vi "Dashboard Main.vi"() -> ()   [LabVIEW 2012]
uses:
  <vilib>/Utility/config.llb/Read Key (String).vi
  <vilib>/Utility/config.llb/Read Key (I32).vi
  <vilib>/Utility/config.llb/Write Key (String).vi
  <vilib>/Utility/config.llb/Write Key (I32).vi
  <vilib>/Utility/config.llb/NI_LVConfig.lvlib
panel:
  in  "?":bool
  out "Camera Image 2":T1(plugin-control)
  out "Mbps":dbl format="%#.1g"
  in  "Enable":bool
  in  "DB Camera Config":bool
  out "Mbps 2":bool
  out "fps":dbl format="%#.1g"
  out "Camera Image":T1(plugin-control)
  out "Battery Value":dbl(slide) scale=0.0..14.0 scale format="%#_2e"
  out "Battery":sgl(graph)
  in  "Camera Settings":T2={"Frate Rate"=30, "Compression"=30, "Size"=1} {"Frate Rate" scale=1.0..30.0; "Size" items=["640x480", "320x240", "160x120"]}
  out "Mode":T3(ring)=enum."Auto Disabled"
  out "Robot IP":string
  # "Robot IP:"
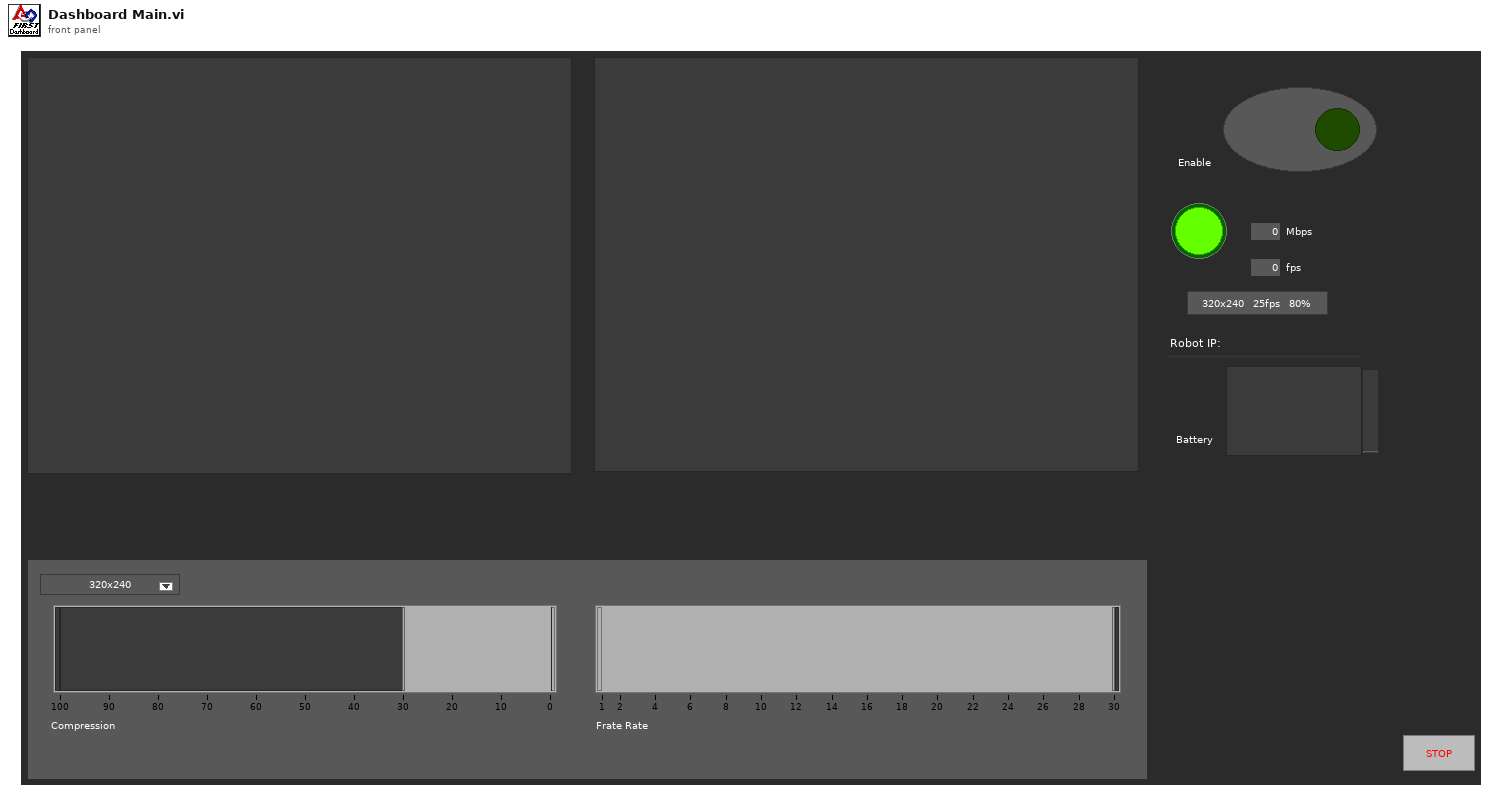
[diagram p1: front panel]
types:
  T1 = typedef "IMAQ Image.ctl" = refnum<image>
  T2 = cluster{"Frate Rate":i32, "Compression":i32, "Size":u16}
  T3 = enum8{"Tele-Op Disabled", "Tele-Op Enabled", "Auto Disabled", "Auto Enabled", "Test Disabled", "Test Enabled", ""}
  T4 = typedef "Image Type" = u32
  T5 = typedef "LVRectTypeDef.ctl" = cluster{"Left":i16, "Top":i16, "Right":i16, "Bottom":i16}
  T6 = cluster{"Competition mode":bool, "Robot Link":bool, "Autonomous":bool, "Enabled":bool, "E-Stop":bool, "Simulated":bool, "TestMode":bool, "Docked Window":bool}
  T7 = typedef "NI_LVConfig.lvlib/Config Data RefNum.ctl" = refnum<k1>
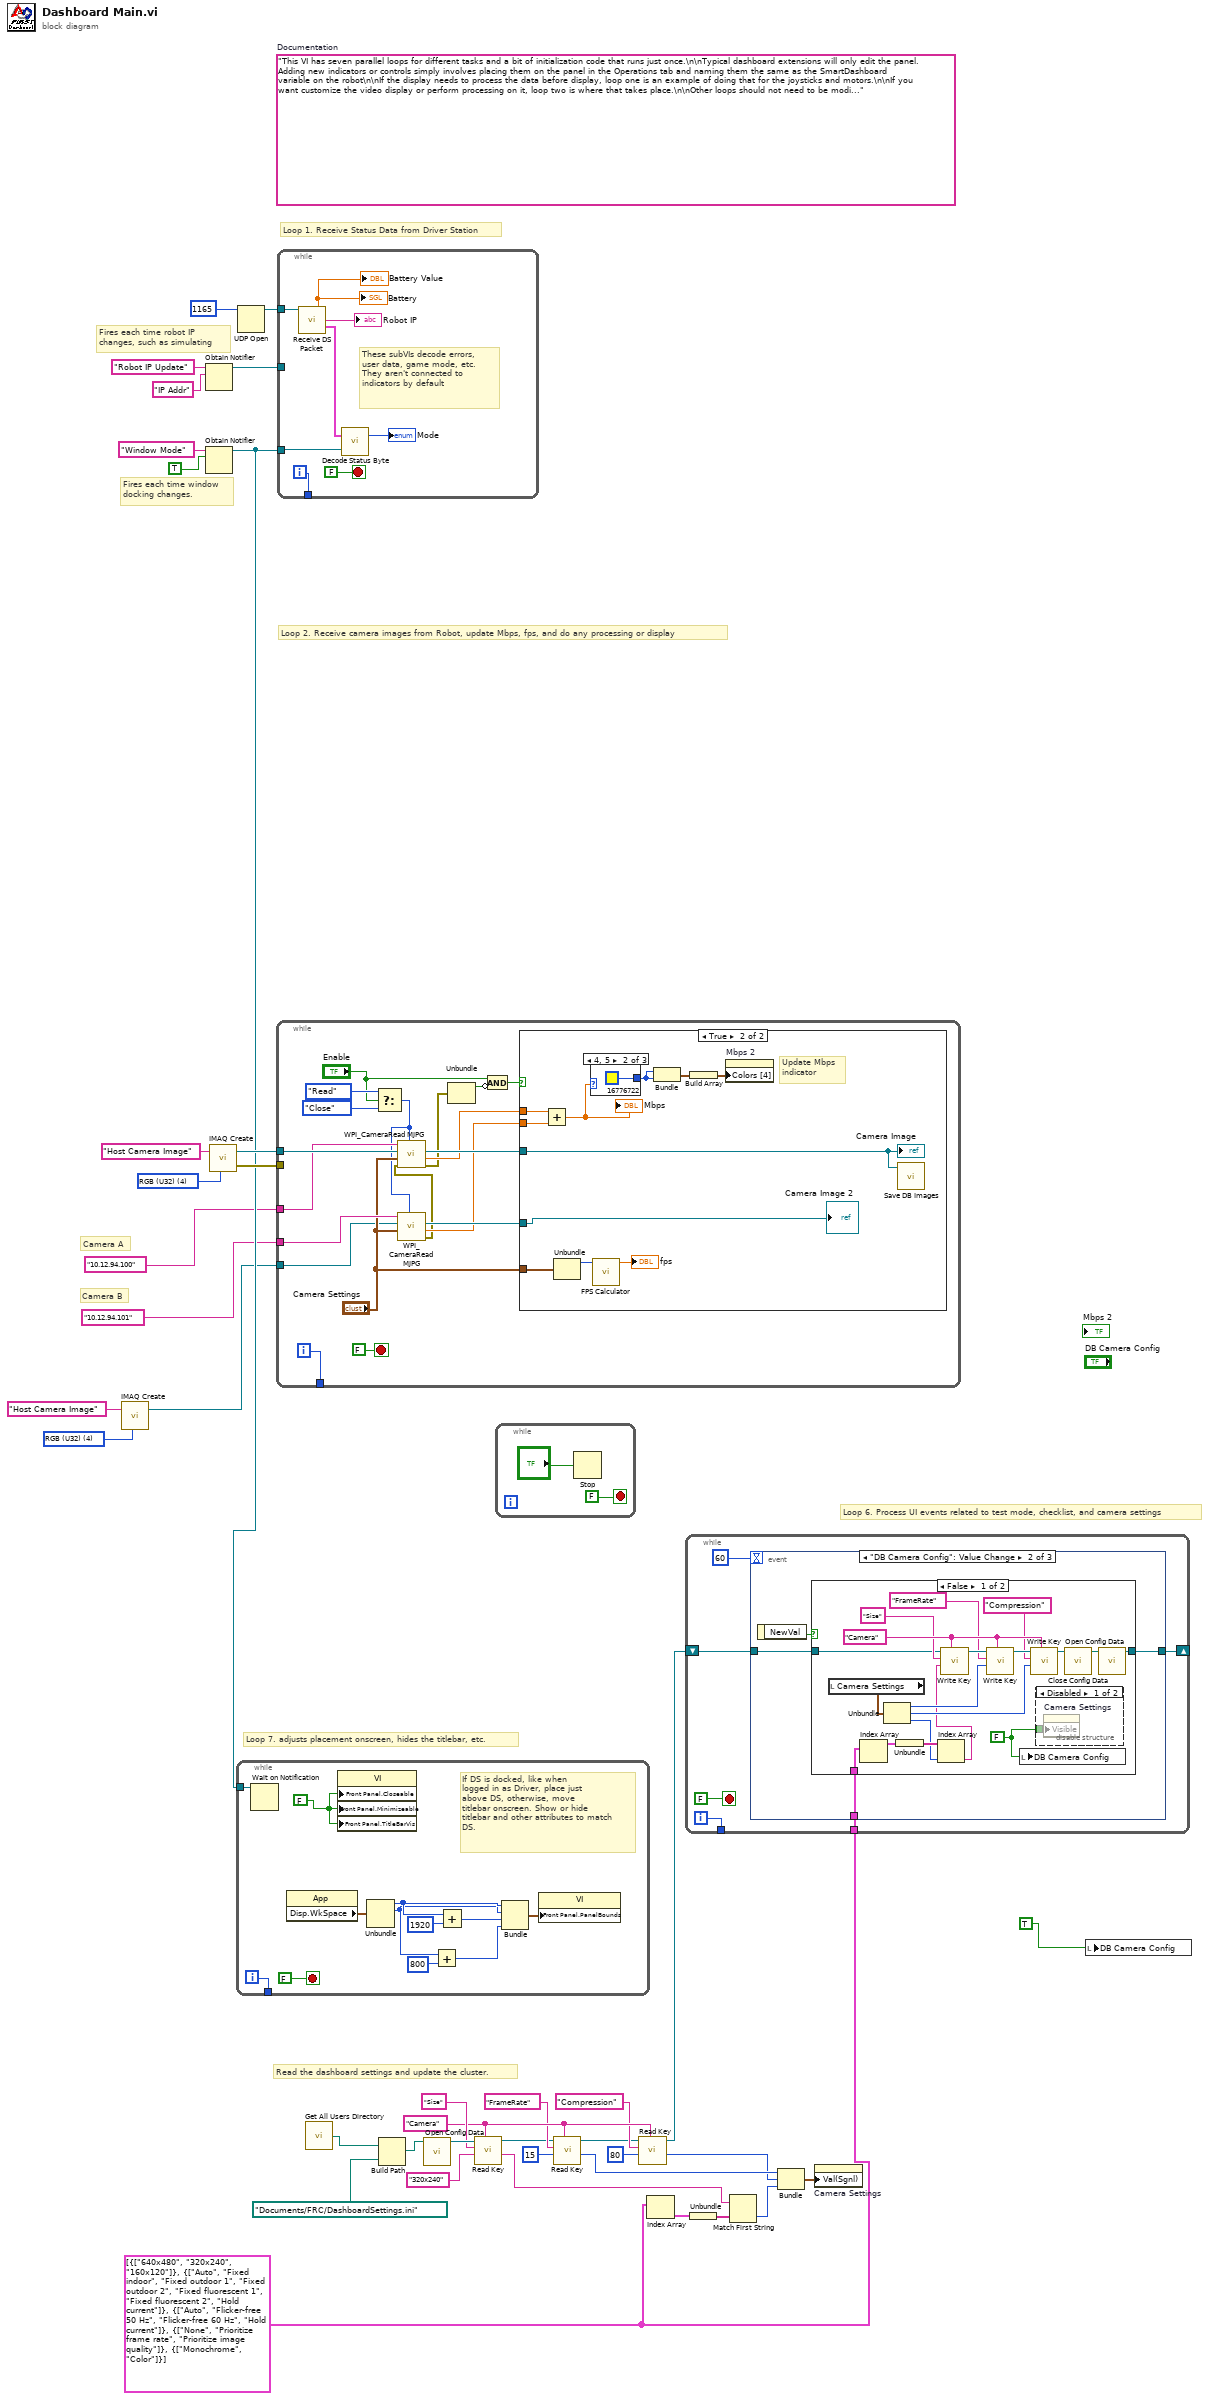
[diagram p0: block diagram]
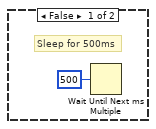
[diagram p2: hidden frame]
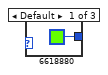
[diagram p3: hidden frame]
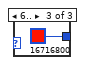
[diagram p4: hidden frame]
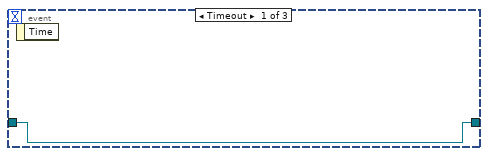
[diagram p5: hidden frame]
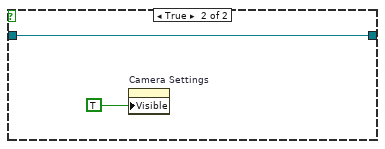
[diagram p7: hidden frame]
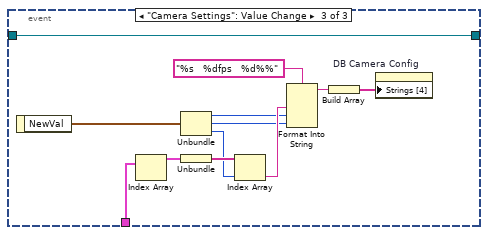
[diagram p8: hidden frame]
diagram:
  w3 = T4 4 items=["Grayscale (U8)", "Grayscale (I16)", "Grayscale (SGL)", "Complex (CSG)", "RGB (U32)", "HSL (U32)", "RGB (U64)"] ("Image Type")
  w22 = "Camera"
  w14 = cluster{string[]}[] [{["640x480", "320x240", "160x120"]}, {["Auto", "Fixed indoor", "Fixed outdoor 1", "Fixed outdoor 2", "Fixed fluorescent 1", "Fixed fluorescent 2", "Hold current"]}, {["Auto", "Flicker-free 50 Hz", "Flicker-free 60 Hz", "Hold current"]}, {["None", "Prioritize frame rate", "Prioritize image quality"]}, {["Monochrome", "Color"]}]
  (unwired) "This VI has seven parallel loops for different tasks and a bit of initialization code that runs just once.\n\nTypical dashboard extensions will only edit the panel. Adding new indicators or controls simply involves placing them on the panel in the Operations tab and naming them the same as the SmartDashboard variable on the robot\n\nIf the display needs to process the data before display, loop one is an example of doing that for the joysticks and motors.\n\nIf you want customize the video display or perform processing on it, loop two is where that takes place.\n\nOther loops should not need to be modified. They are pretty standard, and document the task they perform."  # Documentation
  w38 = T4 4 items=["Grayscale (U8)", "Grayscale (I16)", "Grayscale (SGL)", "Complex (CSG)", "RGB (U32)", "HSL (U32)", "RGB (U64)"] ("Image Type")
  # "Camera B"
  # "Camera A"
  # "Fires each time robot IP\nchanges, such as simulating"
  # "Fires each time window\ndocking changes."
  # "Loop 6. Process UI events related to test mode, checklist, and camera settings"
  # "Read the dashboard settings and update the cluster."
  # "Loop 7. adjusts placement onscreen, hides the titlebar, etc."
  # "Loop 1. Receive Status Data from Driver Station"
  # "Loop 2. Receive camera images from Robot, update Mbps, fps, and do any processing or display"
  n1 = call "IMAQ Create"("Image Name"="Host Camera Image", "Image Type"=w3) -> ("New Image"=w1:T1)  [unwired: 2 in, 2 out]
  n2 = Obtain Notifier(name (unnamed)="Robot IP Update", notification data type="IP Addr" ("name (unnamed)")) -> (notifier out=w32:refnum<notifier>)  [unwired: 2 in, 2 out]
  n3 = Obtain Notifier(name (unnamed)="Window Mode", notification data type=TRUE) -> (notifier out=w29:refnum<notifier>)  [unwired: 2 in, 2 out]
  n4 = call "IMAQ Create"("Image Name"="Host Camera Image", "Image Type"=w38) -> ("New Image"=w36:T1, "error out"=w35:errorcluster)  [unwired: 2 in, 1 out]
  n5 = while {
    tunnel: w29 -> [w51]
    tunnel: [w50] -> _
    i -> [w50]
    stop <- FALSE stop-if-true
    w41 = FALSE ("Front Panel Window:Closeable")
    # "If DS is docked, like when\nlogged in as Driver, place just\nabove DS, otherwise, move\ntitlebar onscreen. Show or hide\ntitlebar and other attributes to match\nDS."
    n6 = Wait on Notification(notifier=w51) -> ()  [unwired: 3 in, 4 out]
    n7 = property class="App"() -> ("Disp.WkSpace"=w43:T5)  [unwired: 2 in, 2 out]
    n8 = property class="VI"("Front Panel.Closeable"=w41, "Front Panel.Minimizeable"=w41, "Front Panel.TitleBarVis"=w41) -> ()  [unwired: 2 in, 2 out]
    n9 = Unbundle(w43) -> ("Left"=w49:i16, "Top"=w48:i16)  [unwired: 2 out]
    n10 = Add(x=w48, y=i16 800) -> (x+y=w45:i16)
    n11 = Add(x=w49, y=i16 1920) -> (x+y=w44:i16)
    n12 = Bundle("Left"=w49, "Top"=w48, w44, w45) -> (w42:cluster{"Left":i16, "Top":i16, i16, i16})  [unwired: 1 out]
    n13 = property class="VI"("Front Panel.PanelBounds"=w42) -> ()  [unwired: 2 in, 2 out]
  }
  n14 = UDP Open(11:u16 1165 ("port")) -> (port=w39:refnum<k16>)  [unwired: 2 in, 4 out]
  n15 = while {
    tunnel: w36 -> [w69]
    tunnel: w35 -> [_]
    tunnel: [w70] -> _
    tunnel: "10.12.94.100" -> [w56]
    tunnel: "10.12.94.101" -> [w58]
    tunnel: w1 -> [w55]
    i -> [w70]
    stop <- FALSE stop-if-true
    n16 = Select(t=enum16{"Read", "Reopen", "Close"}."Read" ("Operation"), s="Enable", f=enum16{"Read", "Reopen", "Close"}."Close" ("Operation")) -> (s? t:f=w53:enum16{"Read", "Reopen", "Close"})
    n17 = call <vilib>:"WPI_CameraRead MJPG.vi"("Operation"=w53, "Camera Settings"="Camera Settings", "Image"=w55, "address"=w58) -> ("error out"=w54:errorcluster, "Bandwidth (kbps)"=w59:dbl, "Image Out"=w60:T1)  [unwired: 5 in]
    n18 = call <vilib>:"WPI_CameraRead MJPG.vi"("Operation"=w53, "error in"=w54, "Camera Settings"="Camera Settings", "Image"=w69, "address"=w56) -> ("error out"=w64:errorcluster, "Bandwidth (kbps)"=w67:dbl, "Image Out"=w68:T1)  [unwired: 4 in]
    n19 = Unbundle(w64) -> ("status"=w62:bool)  [unwired: 2 out]
    n20 = Compound Arithmetic op=AND("Enable", invert w62) -> (w61:bool)
    n21 = case shown="True" w61 {
      tunnel: "Camera Settings" -> [_ w79]
      tunnel: w68 -> [_ w77]
      tunnel: w67 -> [_ w75]
      tunnel: w60 -> [_ w73]
      tunnel: w59 -> [_ w76]
      frame False {
        # "Sleep for 500ms"
        n22 = Wait Until Next ms Multiple(millisecond multiple=u32 500) -> ()  [unwired: 1 out]
      }
      frame True {
        # "Update Mbps\nindicator"
        n23 = Add(x=w75, y=w76) -> (x+y=w74:dbl)
        "Mbps" <- w74
        n24 = Unbundle(w79) -> ("Frate Rate"=w78:i32)  [unwired: 2 out]
        n25 = case shown="4, 5" w74 {
          tunnel: [u32 6618880 ("Color Box") u32 16776722 ("Color Box") u32 16716800 ("Color Box")] -> w81
          frame Default {
          }
          frame 4, 5 {
          }
          frame 6.. {
          }
        }
        n26 = call "FPS Calculator.vi"("Average Count"=w78) -> ("fps"=→"fps":dbl)  [unwired: 10 in]
        n27 = Bundle("Color Box"=w81, "Color Box"=w81) -> (w83:cluster{"Color Box":u32, "Color Box":u32})  [unwired: 1 out]
        n28 = Build Array(w83) -> (w82:cluster{"Color Box":u32, "Color Box":u32}[])
        n29 = property on="Mbps 2" class="Bool (strict)"("Colors [4]"=w82) -> ()  [unwired: 2 in, 2 out]
        n30 = call "Save DB Images.vi"("Image"=w77) -> ()  [unwired: 2 in, 1 out]
        "Camera Image" <- w77
        "Camera Image 2" <- w73
      }
    }
  }
  n31 = while {
    tunnel: w39 -> [w92]
    tunnel: w32 -> [_]
    tunnel: w29 -> [w90]
    tunnel: [w88] -> _
    i -> [w88]
    stop <- FALSE stop-if-true
    # "These subVIs decode errors, user data, game mode, etc.\nThey aren't connected to indicators by default"
    n32 = call "Receive DS Packet.vi"("Recv Socket"=w92) -> ("Battery"=→"Battery" →"Battery Value":sgl, "Robot IP Address"=→"Robot IP":string, "Status"=w93:T6)  [unwired: 1 in, 11 out]
    n33 = call "Decode Status Byte.vi"("Window Mode Notifier"=w90, "Status"=w93) -> ("Mode"=→"Mode":T3)  [unwired: 1 out]
  }
  n34 = call "Get All Users Directory.vi"() -> ("All User Path"=w27:path)
  n35 = Build Path(base path=w27, name or relative path=path "Documents/FRC/DashboardSettings.ini") -> (appended path=w26:path)
  n36 = call <vilib>:"Open Config Data.vi"("configuration file path"=w26) -> ("refnum"=w25:T7)  [unwired: 8 in, 2 out]
  n37 = call-poly <vilib>:"Read Key.vi"("section"=w22, "default value"="320x240", "key"="Size", "refnum"=w25) -> ("value"=w12:string, "refnum out"=w9:T7)  [unwired: 2 in, 4 out]
  n38 = while {
    stop <- FALSE stop-if-true
    n39 = Stop(stop? (T)="?") -> ()
  }
  n40 = call-poly <vilib>:"Read Key.vi"("section"=w22, "default value"=15, "key"="FrameRate", "refnum"=w9) -> ("value"=w17:i32, "refnum out"=w8:T7)  [unwired: 1 in, 5 out]
  n41 = call-poly <vilib>:"Read Key.vi"("section"=w22, "default value"=80, "key"="Compression", "refnum"=w8) -> ("value"=w16:i32, "refnum out"=w6:T7)  [unwired: 1 in, 5 out]
  n42 = Index Array(array=w14) -> (element=w15:cluster{string[]})  [unwired: 1 in]
  n43 = while {
    tunnel: w14 -> [w100]
    shift-right: [w99] -> _
    shift-left: w6 -> [w98]
    tunnel: [w97] -> _
    i -> [w97]
    stop <- FALSE stop-if-true
    n44 = event shown="[1] \"DB Camera Config\": Value Change" {
      selector: _ -> [_ _ _]
      dyn-events: _ -> [_ _ _]
      timeout: u32 60 ("milliseconds to wait") -> [_ _ _]
      tunnel: w100 -> [_ w106 w137]
      tunnel: [w103 w105 w130] -> w99
      tunnel: w98 -> [w103 w104 w130]
      event Timeout {
        n45 = event-data() -> ()  [unwired: 1 in, 1 out]
      }
      event "DB Camera Config": Value Change {
        n46 = event-data() -> ("NewVal"=w107:bool)  [unwired: 1 in]
        n47 = case shown="False" w107 {
          tunnel: w106 -> [w116 _]
          tunnel: [w109 w128] -> w105
          tunnel: w104 -> [w108 w128]
          frame False {
            w123 = "Camera"
            w126 = FALSE ("Visible")
            n48 = local read "Camera Settings"() -> (w115:T2)
            n49 = Index Array(array=w116) -> (element=w119:cluster{string[]})  [unwired: 1 in]
            n50 = Unbundle(w115) -> ("Frate Rate"=w114:i32, "Compression"=w113:i32, "Size"=w117:u16)
            n51 = Unbundle(w119) -> (w118:string[])
            n52 = Index Array(array=w118, index=w117) -> (element=w112:string)
            n53 = call-poly <vilib>:"Write Key.vi"("section"=w123, "value"=w112, "key"="Size", "refnum"=w108) -> ("refnum out"=w125:T7)  [unwired: 2 in, 5 out]
            n54 = call-poly <vilib>:"Write Key.vi"("section"=w123, "value"=w114, "key"="FrameRate", "refnum"=w125) -> ("refnum out"=w124:T7)  [unwired: 1 in, 6 out]
            n55 = local write "DB Camera Config"(w126) -> ()
            n56 = call-poly <vilib>:"Write Key.vi"("section"=w123, "value"=w113, "key"="Compression", "refnum"=w124) -> ("refnum out"=w110:T7)  [unwired: 1 in, 6 out]
            n57 = disable-structure shown="Disabled" {
              disable-tunnel: w126 -> [w127 _]
              frame Disabled {
                n58 = property on="Camera Settings" class="Clust (strict)"("Visible"=w127) -> ()  [unwired: 2 in, 2 out]
              }
              frame Enabled {
              }
            }
            n59 = call <vilib>:"Close Config Data.vi"("refnum"=w110) -> ("file path"=w111:path)  [unwired: 2 in, 8 out]
            n60 = call <vilib>:"Open Config Data.vi"("configuration file path"=w111) -> ("refnum"=w109:T7)  [unwired: 8 in, 2 out]
          }
          frame True {
            n61 = property on="Camera Settings" class="Clust (strict)"("Visible"=TRUE) -> ()  [unwired: 2 in, 2 out]
          }
        }
      }
      event "Camera Settings": Value Change {
        n62 = event-data() -> ("NewVal"=w141:T2)  [unwired: 1 in]
        n63 = Index Array(array=w137) -> (element=w136:cluster{string[]})  [unwired: 1 in]
        n64 = Unbundle(w141) -> ("Frate Rate"=w132:i32, "Compression"=w131:i32, "Size"=w134:u16)
        n65 = Unbundle(w136) -> (w135:string[])
        n66 = Index Array(array=w135, index=w134) -> (element=w133:string)
        n67 = Format Into String(format string="%s   %dfps   %d%%", w133, w132, w131) -> (resulting string=w138:string)  [unwired: 2 in, 1 out]
        n68 = Build Array(w138) -> (w139:string[])
        n69 = property on="DB Camera Config" class="Bool (strict)"("Strings [4]"=w139) -> ()  [unwired: 2 in, 2 out]
      }
    }
  }
  n70 = Unbundle(w15) -> (w13:string[])
  n71 = Match First String(2:w13, 3:w12) -> (0:w11:i32)  [unwired: 1 out]
  n72 = Bundle("value"=w17, "value"=w16, "index"=w11) -> (w7:cluster{"value":i32, "value":i32, "index":i32})  [unwired: 1 out]
  n73 = property on="Camera Settings" class="Clust (strict)"("Val(Sgnl)"=w7) -> ()  [unwired: 2 in, 2 out]
  n74 = local write "DB Camera Config"(TRUE ("Visible")) -> ()
